vi "AMI_SetTemperature.vi"(6 "error in (no error)":errorcluster, 7 "Index":i8) -> (0 "error out":errorcluster, 2 "resulting string 1":string="Set Temperatura 4.2K at 20K/min, FastSettle, Sweep&meas", 3 "Cancelled?":bool)   [LabVIEW 2017]
doc: "Use this template to create a dialog box. This template polls the state of the buttons on the front panel and does not use events. Use the Dialog Using Events template (not available in Base package) to create a dialog box with event handling."
panel:
  out "Wait stability":bool=TRUE
  in  "Approach":i32(ring) items=["FastSettle", "NoOvershoot"]
  in  "Rate (K/min)":dbl=20.0
  in  "Temperatura (K)":dbl=4.2
  in  "Cancel":bool
  in  "OK":bool
  # "SET TEMPERATURE"
  # "Enero 2023 V1.3  a-sslcdms"
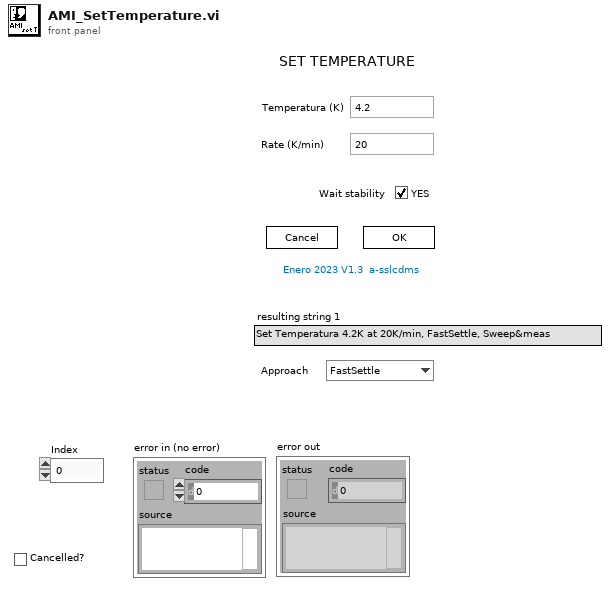
[diagram p1: front panel]
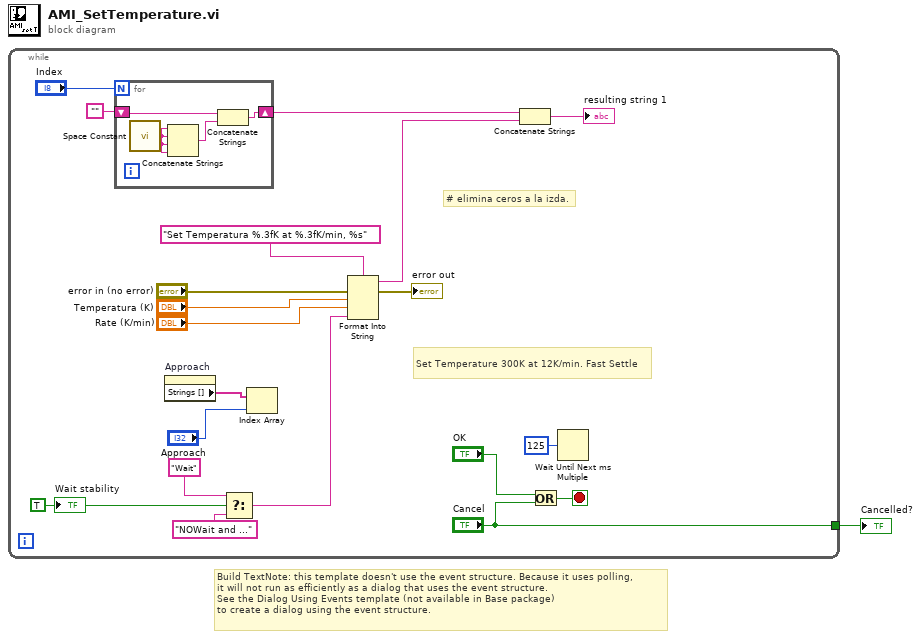
[diagram p0: block diagram]
diagram:
  # "Build TextNote: this template doesn't use the event structure. Because it uses polling, \nit will not run as efficiently as a dialog that uses the event structure.\nSee the Dialog Using Events template (not available in Base package) \nto create a dialog using the event structure."
  n1 = while {
    tunnel: ["Cancel"] -> w1
    stop <- w20 stop-if-true
    w4 = TRUE ("Wait stability")
    # "Set Temperature 300K at 12K/min. Fast Settle"
    # "# elimina ceros a la izda."
    n2 = for {
      N: "Index" -> [_]
      shift-right: [w24] -> w10
      shift-left: "" -> [w23]
      n3 = call <vilib>:"Space Constant.vi"() -> ("String"=w22:string)
      n4 = Concatenate Strings(w22, w22, w22, w22) -> (w25:string)
      n5 = Concatenate Strings(w23, w25) -> (w24:string)
    }
    n6 = property on="Approach" class="Ring (strict)"() -> ("Strings []"=w9:string[])  [unwired: 2 in, 2 out]
    n7 = Select(t="Wait", s=w4, f="NOWait and ...") -> (s? t:f=w2:string)
    n8 = Index Array(array=w9, index="Approach") -> ()  [unwired: 1 out]
    n9 = Format Into String(format string="Set Temperatura %.3fK at %.3fK/min, %s", error in="error in (no error)", "Temperatura (K)", "Rate (K/min)", w2) -> (resulting string=w12:string, error out=→"error out":errorcluster)  [unwired: 1 in]
    n10 = Concatenate Strings(w10, w12) -> (→"resulting string 1":string)
    n11 = Or(x="OK", y="Cancel") -> (x .or. y?=w20:bool)
    n12 = Wait Until Next ms Multiple(millisecond multiple=u32 125) -> ()  [unwired: 1 out]
    "Wait stability" <- w4
  }
  "Cancelled?" <- w1
